vi "BSON_bytes_to_I64.vi"(11 "BSONbytes":u8[](array[numeric])) -> (3 "value":i64)   [LabVIEW 2015, in "BSON_convertors_Library.lvlib"]
uses:
  BSON_convertors_Library.lvlib
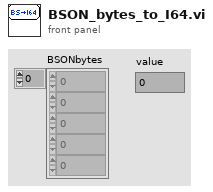
[diagram p1: front panel]
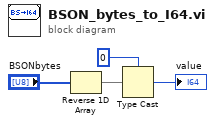
[diagram p0: block diagram]
diagram:
  n1 = Reverse 1D Array(array="BSONbytes") -> (reversed array=w3:u8[])
  n2 = Type Cast(type=i64 0, x=w3) -> (*(type *) &x=→"value":i64)
